vi "mono_start_sensor_stream.vi"(4 "error in":errorcluster, 5 "TCP Network Connection in":refnum<k5>, 6 "stream_command_cluster":T1) -> (0 "error out":errorcluster, 1 "TCP Network Connection out":refnum<k5>, 3 "stream response":string)   [LabVIEW 2018]
uses:
  mono_commands.ctl
panel:
  out "JSON string":string
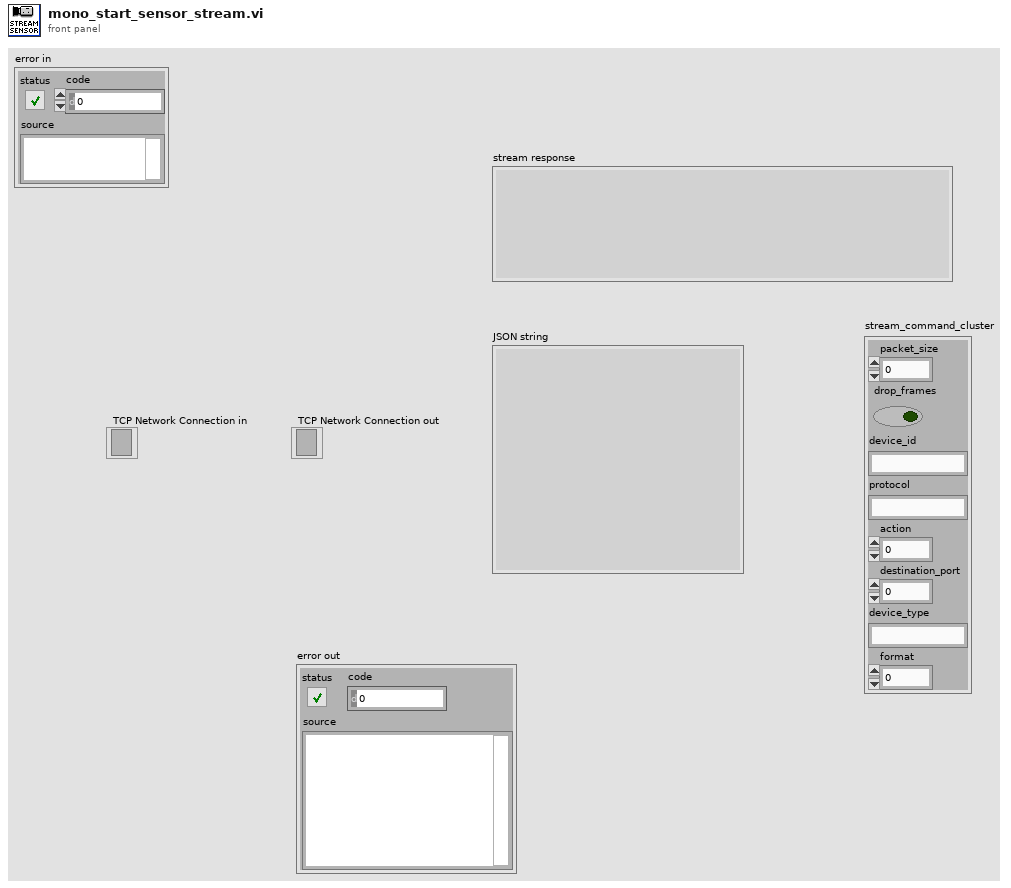
[diagram p1: front panel]
types:
  T1 = cluster{"packet_size":i32, "drop_frames":bool, "device_id":string, "protocol":string, "action":i32, "destination_port":i32, "device_type":string, "format":i32}
  T2 = cluster{"class":string, "status":u32, "messages":string[], "data":cluster{"packet_size":i32, "drop_frames":bool, "device_id":string, "protocol":string, "action":i32, "destination_port":i32, "device_type":string, "format":i32}}
  T3 = typedef "mono_commands.ctl" = cluster{"SIMULATOR_STATUS_UUID":string, "STREAM_DATA_COMMAND_UUID":string, "SIMULATOR_CONFIG_COMMAND_UUID":string, "VEHICLE_CONFIG_COMMAND_UUID":string, "EGO_CONTROL_COMMAND_UID":string, "WAYPOINT_UPDATE_COMMAND_UID":string, "SCENARIO_COMMAND_UID":string, "MAP_COMMAND_UID":string, "SPAWN_COMMAND_UID":string, "MOVE_ACTOR_COMMAND_UID":string, "SCENARIO_INIT_COMMAND_UID":string, "ATTACH_SENSOR_COMMAND_UID":string, "DETACH_SENSOR_COMMAND_UID":string, "CONTROL_HEADER":string, "RESPONSE_HEADER":string}
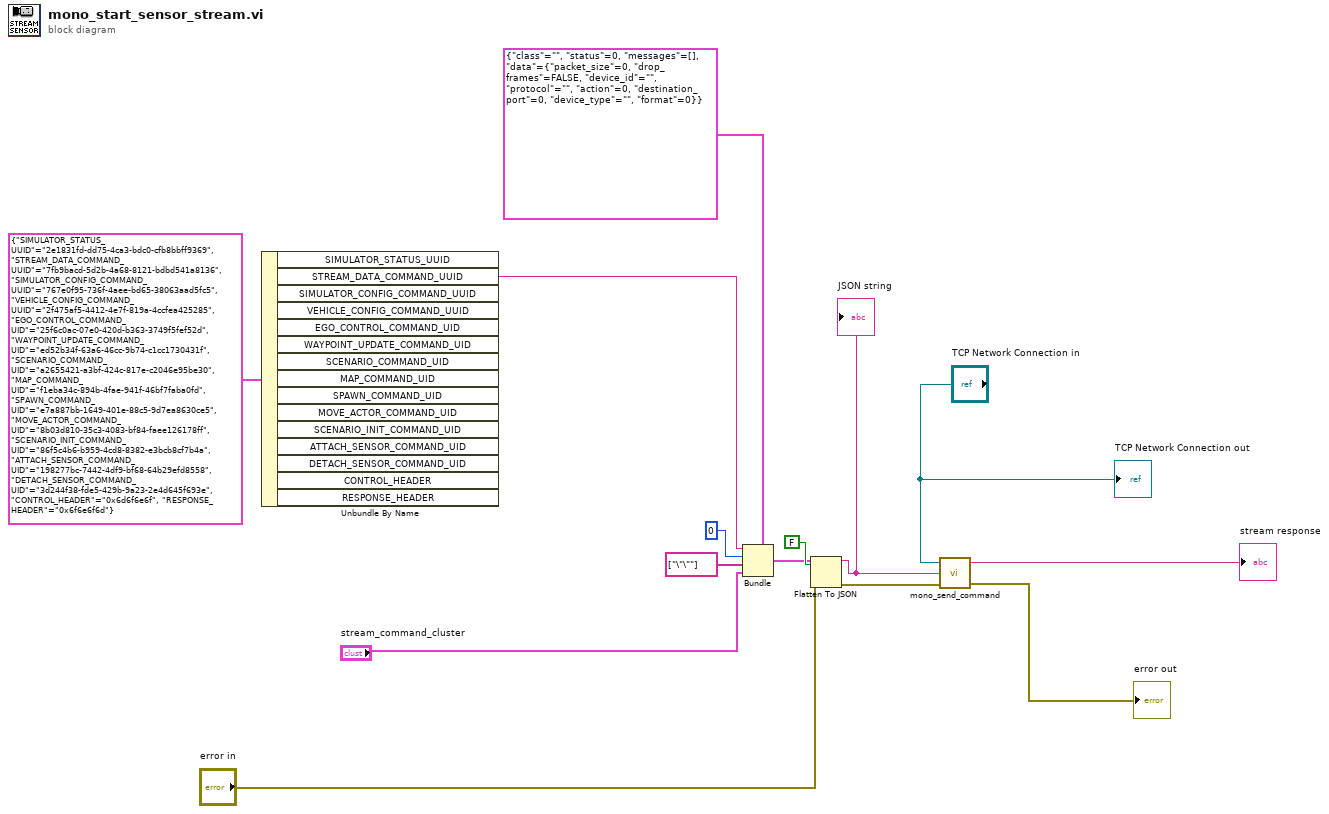
[diagram p0: block diagram]
diagram:
  n1 = Unbundle By Name(T3 {"SIMULATOR_STATUS_UUID"="2e1831fd-dd75-4ca3-bdc0-cfb8bbff9369", "STREAM_DATA_COMMAND_UUID"="7fb9bacd-5d2b-4a68-8121-bdbd541a8136", "SIMULATOR_CONFIG_COMMAND_UUID"="767e0f95-736f-4aee-bd65-38063aad5fc5", "VEHICLE_CONFIG_COMMAND_UUID"="2f475af5-4412-4e7f-819a-4ccfea425285", "EGO_CONTROL_COMMAND_UID"="25f6c0ac-07e0-420d-b363-3749f5fef52d", "WAYPOINT_UPDATE_COMMAND_UID"="ed52b34f-63a6-46cc-9b74-c1cc1730431f", "SCENARIO_COMMAND_UID"="a2655421-a3bf-424c-817e-c2046e95be30", "MAP_COMMAND_UID"="f1eba34c-894b-4fae-941f-46bf7faba0fd", "SPAWN_COMMAND_UID"="e7a887bb-1649-401e-88c5-9d7ea8630ce5", "MOVE_ACTOR_COMMAND_UID"="8b03d810-35c3-4083-bf84-faee126178ff", "SCENARIO_INIT_COMMAND_UID"="86f5c4b6-b959-4cd8-8382-e3bcb8cf7b4a", "ATTACH_SENSOR_COMMAND_UID"="198277bc-7442-4df9-bf68-64b29efd8558", "DETACH_SENSOR_COMMAND_UID"="3d244f38-fde5-429b-9a23-2e4d645f693e", "CONTROL_HEADER"="0x6d6f6e6f", "RESPONSE_HEADER"="0x6f6e6f6d"} ("Cluster")) -> ("STREAM_DATA_COMMAND_UUID"=w1:string)  [unwired: 14 out]
  n2 = Bundle(cluster=T2 {"class"="", "status"=0, "messages"=[], "data"={"packet_size"=0, "drop_frames"=FALSE, "device_id"="", "protocol"="", "action"=0, "destination_port"=0, "device_type"="", "format"=0}}, "class"=w1, "status"=u32 0, "messages"=string[] ["\"\""], "data"="stream_command_cluster") -> (w7:T2)
  n3 = Flatten To JSON(enable LabVIEW extensions? (T)=FALSE, anything=w7, error in (no error)="error in") -> (JSON string=w8:string, 11:w14:errorcluster)
  "JSON string" <- w8
  n4 = call "mono_send_command.vi"("error in (no error)"=w14, "JSON Command"=w8, "TCP Network Connection in"="TCP Network Connection in") -> ("error out"=→"error out":errorcluster, "response"=→"stream response":string)  [unwired: 1 in]
  "TCP Network Connection out" <- "TCP Network Connection in"
